vi "Main.vi"   [LabVIEW 2014]
uses:
  CSV/CSV.lvclass
  Report/Report.lvclass
  TXT/TXT.lvclass
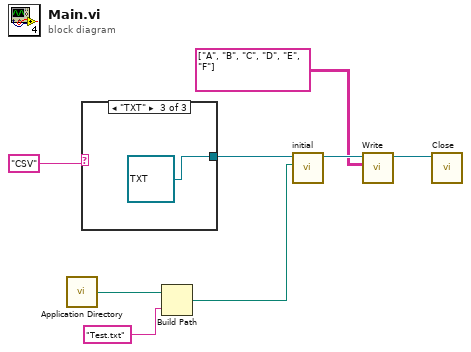
[diagram p0: block diagram]
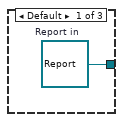
[diagram p2: hidden frame]
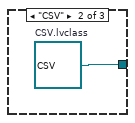
[diagram p3: hidden frame]
diagram:
  n1 = call <vilib>:"Application Directory.vi"() -> ("Application Directory"=w3:path)
  n2 = case shown="\"TXT\"" "CSV" {
    tunnel: [w9 w10 refnum<class "TXT.lvclass"> refnum ("TXT.lvclass")] -> w5
    frame Default {
      w9 = refnum<class "Report.lvclass"> refnum  # Report in
    }
    frame "CSV" {
      w10 = refnum<class "CSV.lvclass"> refnum  # CSV.lvclass
    }
    frame "TXT" {
    }
  }
  n3 = Build Path(base path=w3, name or relative path="Test.txt") -> (appended path=w4:path)
  n4 = call-dynamic "initial.vi"("Path"=w4, "Report in"=w5) -> ("Report out"=w8:refnum<class "Report.lvclass">)  [unwired: 8 in, 1 out]
  n5 = call-dynamic "Write.vi"("Array"=string[][] [["A", "B", "C"], ["D", "E", "F"]], "Report in"=w8) -> ("Report out"=w7:refnum<class "Report.lvclass">)  [unwired: 8 in, 1 out]
  n6 = call-dynamic "Close.vi"("Report in"=w7) -> ()  [unwired: 9 in, 2 out]
